vi "ATF Storage-UI Commands_R.vi"(11 "Data FIFO Ref":T1) -> ()   [LabVIEW 2022 SP3]
doc: "Use this template to build a simple state machine design pattern. Each state executes code and determines which state to transition to."
uses:
  RT Controls/ATF Storage-Data FIFO.ctl
  RT Controls/ATF Storage-NS Enum.ctl
  RT Controls/ATF Storage-Data Type Control screen.ctl
  RT Controls/ATF Storage Haelth.ctl
  RT Support/ATF Storage-RT_Global_R.vi
panel:
  out "Sts":bool
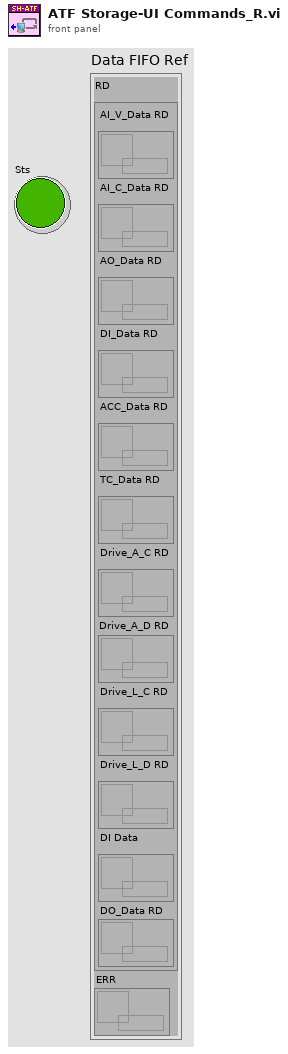
[diagram p1: front panel]
types:
  T1 = typedef "ATF Storage-Data FIFO.ctl" = cluster{"RD":cluster{"AI_V_Data RD":refnum<queue>, "AI_C_Data RD":refnum<queue>, "AO_Data RD":refnum<queue>, "DI_Data RD":refnum<queue>, "ACC_Data RD":refnum<queue>, "TC_Data RD":refnum<queue>, "Drive_A_C RD":refnum<queue>, "Drive_A_D RD":refnum<queue>, "Drive_L_C RD":refnum<queue>, "Drive_L_D RD":refnum<queue>, "DI Data":refnum<queue>, "DO_Data RD":refnum<queue>}, "ERR":refnum<queue>}
  T2 = cluster{"Reader":refnum<k21>, "Writer":refnum<k21>, "Er":refnum<queue>}
  T3 = typedef "ATF Storage-NS Enum.ctl" = enum16{"Initialize", "Listen for UI Writer", "Send data", "Exit"}
  T4 = typedef "ATF Storage Haelth.ctl" = enum16{"AI C", "AI V", "AO", "DI", "DO", "TC", "ACC", "RT Str", "DR A"}
  T5 = enum16{"Init", "Read 'All'", "Read 'n'", "Read '1'", "Write '1'", "Write 'n'", "Write 'All'"}
  T6 = cluster{"Start DAQ":bool, "Stop DAQ":bool, "RT Stop":bool, "RT Exit":bool, "Start Seq":bool}
  T7 = typedef "ATF Storage-Data Type Control screen.ctl" = cluster{"DI_Data":digitalwaveform[], "Drive_A_C":waveform(dbl)[], "Drive_A_D":waveform(dbl)[], "Drive_L_C":waveform(dbl)[], "Drive_L_D":waveform(dbl)[], "Loop Status":bool[], "CDT Timer":dbl, "RT Error":cluster{"Error Code":string, "Error Source":string}, "DO":waveform(dbl)[], "SEQ Monitor":string[], "Device List":string}
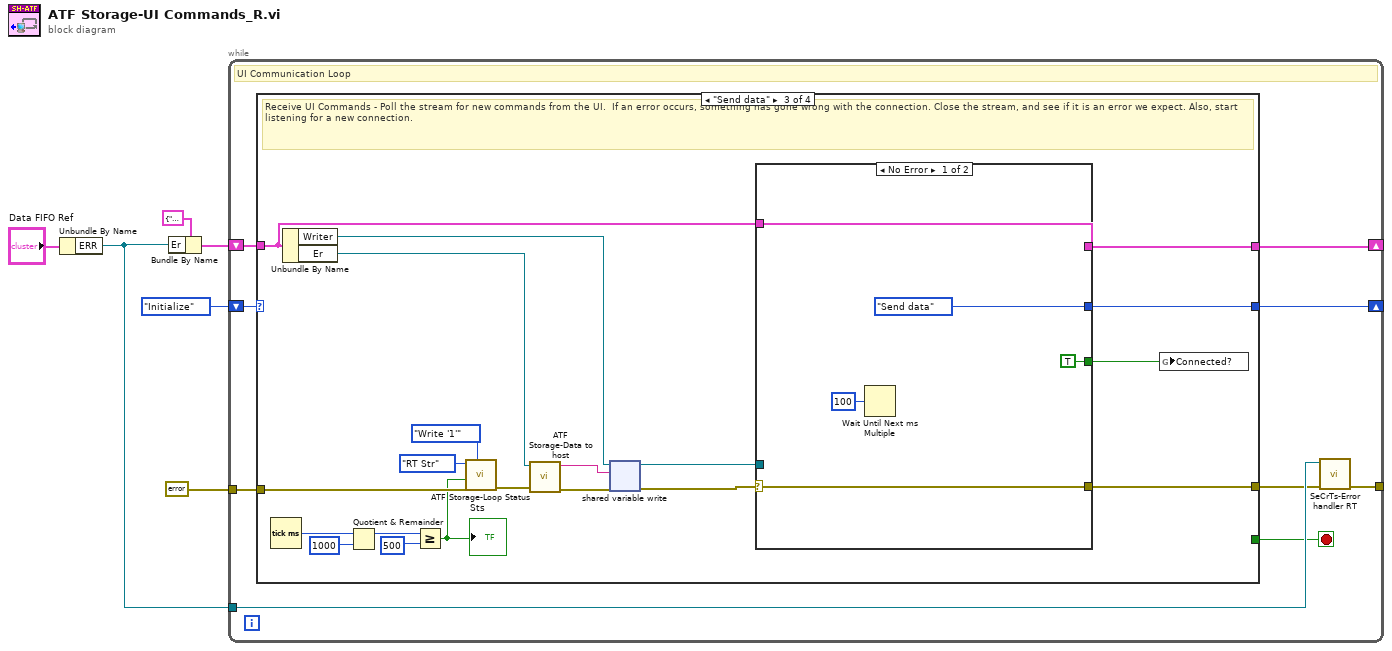
[diagram p0: block diagram]
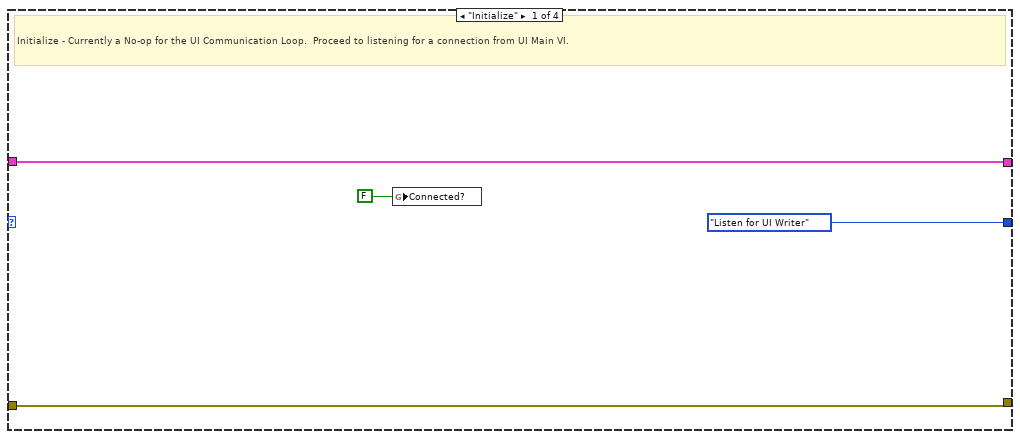
[diagram p2: hidden frame]
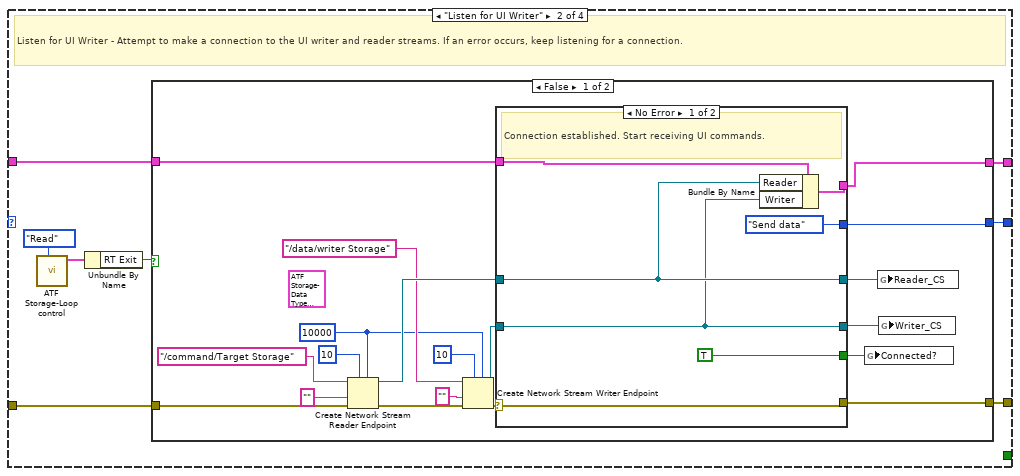
[diagram p3: hidden frame]
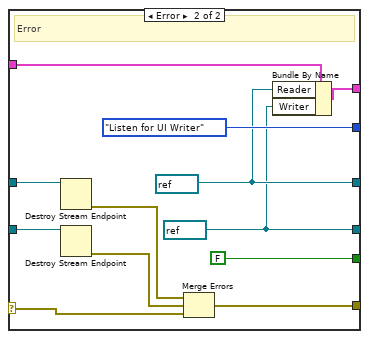
[diagram p4: hidden frame]
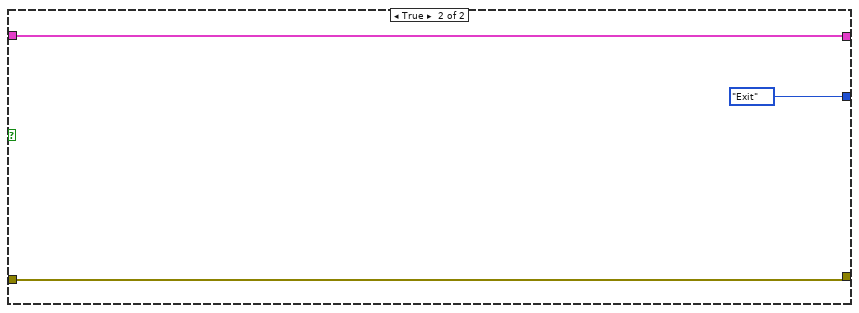
[diagram p5: hidden frame]
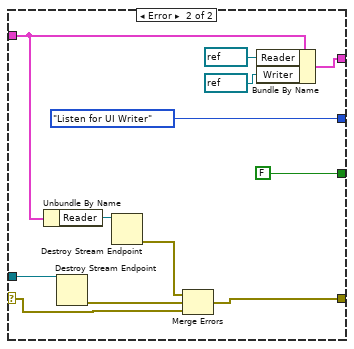
[diagram p6: hidden frame]
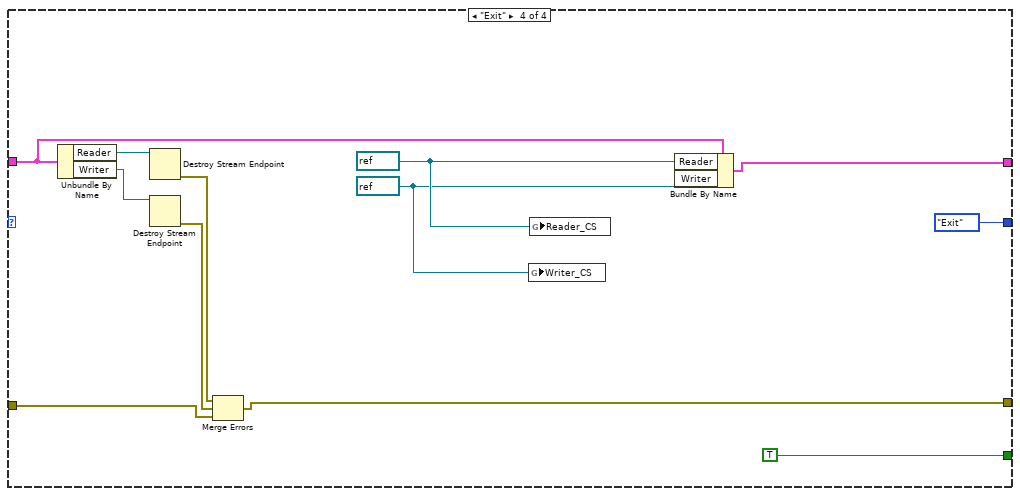
[diagram p7: hidden frame]
diagram:
  n1 = Unbundle By Name("Data FIFO Ref") -> ("ERR"=w1:refnum<queue>)
  n2 = Bundle By Name(cluster=T2 {"Reader"="", "Writer"="", "Er"=refnum}, "Er"=w1) -> (w4:T2)
  n3 = while {
    shift-right: [w14] -> _
    shift-left: ATF_Storage-NS_Enum."Initialize" ("Enum") -> [w15]
    tunnel: w1 -> [w13]
    shift-right: [w9] -> _
    shift-left: w4 -> [w10]
    tunnel: errorcluster {"status"=FALSE, "code"=0, "source"=""} ("error in (no error)") -> [w11]
    tunnel: [w7] -> _
    stop <- w8 stop-if-true
    # "UI Communication Loop"
    n4 = case shown="\"Send data\"" w15 {
      tunnel: [w17 w27 w83 w115] -> w12
      tunnel: [ATF_Storage-NS_Enum."Listen for UI Writer" ("Enum") w26 w84 ATF_Storage-NS_Enum."Exit" ("Enum")] -> w14
      tunnel: w11 -> [w17 w25 w74 w106]
      tunnel: w10 -> [w16 w21 w80 w110]
      tunnel: [w16 w20 w81 w111] -> w9
      tunnel: [_ _ _ TRUE] -> w8
      frame "Initialize" {
        # "Initialize - Currently a No-op for the UI Communication Loop.  Proceed to listening for a connection from UI Main VI."
        n5 = global write "ATF Storage-RT_Global_R.vi" "Connected?"(FALSE ("Connected?")) -> ()
      }
      frame "Listen for UI Writer" {
        # "Listen for UI Writer - Attempt to make a connection to the UI writer and reader streams. If an error occurs, keep listening for a connection."
        n6 = call "ATF Storage-Loop control.vi"("Action"=enum16{"Init", "Write", "Read"}."Read") -> ("Loop Control out"=w23:T6)  [unwired: 9 in, 1 out]
        n7 = Unbundle By Name(w23) -> ("RT Exit"=w22:bool)
        n8 = case shown="False" w22 {
          tunnel: [w31 w66] -> w27
          tunnel: [w40 ATF_Storage-NS_Enum."Exit" ("Enum")] -> w26
          tunnel: w25 -> [w34 w66]
          tunnel: w21 -> [w33 w67]
          tunnel: [w32 w67] -> w20
          frame False {
            w30 = 10000 ("timeout in ms (-1)")
            (unwired) T7 {"DI_Data"=[], "Drive_A_C"=[], "Drive_A_D"=[], "Drive_L_C"=[], "Drive_L_D"=[], "Loop Status"=[], "CDT Timer"=0.0, "RT Error"={"Error Code"="", "Error Source"=""}, "DO"=[], "SEQ Monitor"=[], "Device List"=""}
            n9 = Create Network Stream Reader Endpoint(5:w30, 7:10 ("reader buffer size"), 8:w34, 9:"" ("writer url"), 11:"/command/Target Storage" ("reader name")) -> (0:w45:errorcluster, 3:w46:refnum<k21>)  [unwired: 2 in]
            n10 = Create Network Stream Writer Endpoint(5:w30, 7:10 ("writer buffer size"), 8:w45, 9:"" ("reader url"), 11:"/data/writer Storage" ("RT Stream Name_C")) -> (0:w43:errorcluster, 3:w44:refnum<k21>)  [unwired: 2 in]
            n11 = case shown="No Error" w43 {
              selector: w43 -> [w47 w57]
              tunnel: w46 -> [w49 w65]
              tunnel: w44 -> [w48 w64]
              tunnel: [w49 w55] -> w39
              tunnel: [ATF_Storage-NS_Enum."Send data" ("Enum") ATF_Storage-NS_Enum."Listen for UI Writer" ("Enum")] -> w40
              tunnel: [w48 w54] -> w38
              tunnel: [TRUE ("Connected?") FALSE ("Connected?")] -> w35
              tunnel: w33 -> [w51 w61]
              tunnel: [w50 w60] -> w32
              tunnel: [w47 w56] -> w31
              frame No Error {
                # "Connection established. Start receiving UI commands."
                n12 = Bundle By Name(cluster=w51, "Reader"=w49, "Writer"=w48) -> (w50:T2)
              }
              frame Error {
                w54 = refnum<k21> refnum ("RT Stream Name_C")
                w55 = refnum<k21> refnum ("reader name")
                # "Error"
                n13 = Destroy Stream Endpoint(11:w65) -> (0:w59:errorcluster)  [unwired: 1 in]
                n14 = Destroy Stream Endpoint(11:w64) -> (0:w58:errorcluster)  [unwired: 1 in]
                n15 = Merge Errors(w59, w58, w57) -> (w56:errorcluster)
                n16 = Bundle By Name(cluster=w61, "Reader"=w55, "Writer"=w54) -> (w60:T2)
              }
            }
            n17 = global write "ATF Storage-RT_Global_R.vi" "Connected?"(w35) -> ()
            n18 = global write "ATF Storage-RT_Global_R.vi" "Reader_CS"(w39) -> ()
            n19 = global write "ATF Storage-RT_Global_R.vi" "Writer_CS"(w38) -> ()
          }
          frame True {
          }
        }
      }
      frame "Send data" {
        # "Receive UI Commands - Poll the stream for new commands from the UI.  If an error occurs, something has gone wrong with the connection. Close the stream, and see if it is an error we expect. Also, start listening for a new connection."
        n20 = Tick Count (ms)() -> (millisecond timer value=w78:u32)
        n21 = Unbundle By Name(w80) -> ("Writer"=w87:refnum<k21>, "Er"=w86:refnum<queue>)
        n22 = Quotient & Remainder(x=w78, y=u32 1000) -> (x-y*floor(x/y)=w75:u32)  [unwired: 1 out]
        n23 = Greater Or Equal?(x=w75, y=u32 500) -> (x >= y?=w70:bool)
        "Sts" <- w70
        n24 = call "ATF Storage-Loop Status.vi"("Option"=T5."Write '1'", "error in (no error)"=w74, "Status"=w70, "Loop"=ATF_Storage_Haelth."RT Str") -> ("error out"=w73:errorcluster)  [unwired: 5 in, 2 out]
        n25 = call "ATF Storage-Data to host.vi"("error in (no error)"=w73, "Err"=w86) -> ("error out"=w88:errorcluster, "Data"=w79:string)  [unwired: 8 in]
        n26 = shared-variable-write(w87, w88, w79) -> (w82:refnum<k21>, w85:errorcluster)  [unwired: 1 in, 1 out]
        n27 = case shown="No Error" w85 {
          selector: w85 -> [w91 w101]
          tunnel: [ATF_Storage-NS_Enum."Send data" ("Enum") ATF_Storage-NS_Enum."Listen for UI Writer" ("Enum")] -> w84
          tunnel: [w91 w104] -> w83
          tunnel: w82 -> [_ w100]
          tunnel: [w90 w98] -> w81
          tunnel: w80 -> [w90 w97]
          tunnel: [TRUE ("Connected?") FALSE ("Connected?")] -> w69
          frame No Error {
            n28 = Wait Until Next ms Multiple(millisecond multiple=u32 100) -> ()  [unwired: 1 out]
          }
          frame Error {
            n29 = Unbundle By Name(w97) -> ("Reader"=w99:refnum<k21>)
            n30 = Destroy Stream Endpoint(11:w100) -> (0:w102:errorcluster)  [unwired: 1 in]
            n31 = Destroy Stream Endpoint(11:w99) -> (0:w103:errorcluster)  [unwired: 1 in]
            n32 = Merge Errors(w103, w102, w101) -> (w104:errorcluster)
            n33 = Bundle By Name(cluster=w97, "Reader"=refnum<k21> refnum, "Writer"=refnum<k21> refnum) -> (w98:T2)
          }
        }
        n34 = global write "ATF Storage-RT_Global_R.vi" "Connected?"(w69) -> ()
      }
      frame "Exit" {
        w107 = refnum<k21> refnum ("Writer")
        w108 = refnum<k21> refnum ("Reader")
        n35 = Unbundle By Name(w110) -> ("Reader"=w117:refnum<k21>, "Writer"=w116:refnum<k21>)
        n36 = Destroy Stream Endpoint(11:w117) -> (0:w114:errorcluster)  [unwired: 1 in]
        n37 = Destroy Stream Endpoint(11:w116) -> (0:w113:errorcluster)  [unwired: 1 in]
        n38 = Merge Errors(w114, w113, w106) -> (w115:errorcluster)
        n39 = global write "ATF Storage-RT_Global_R.vi" "Writer_CS"(w107) -> ()
        n40 = global write "ATF Storage-RT_Global_R.vi" "Reader_CS"(w108) -> ()
        n41 = Bundle By Name(cluster=w110, "Reader"=w108, "Writer"=w107) -> (w111:T2)
      }
    }
    n42 = call "SeCrTs-Error handler RT.vi"("error in"=w12, "Message Queue"=w13) -> ("error out"=w7:errorcluster)  [unwired: 8 in, 1 out]
  }
